vi "邮件发送.vi"(9 "收件人":string, 10 "reference输入":refnum<vi>, 11 "Boolean输入":refnum<vi>) -> ()   [LabVIEW 2016]
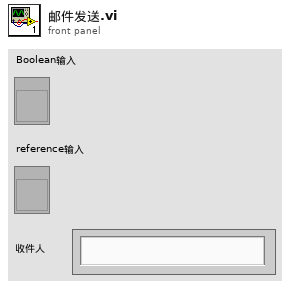
[diagram p1: front panel]
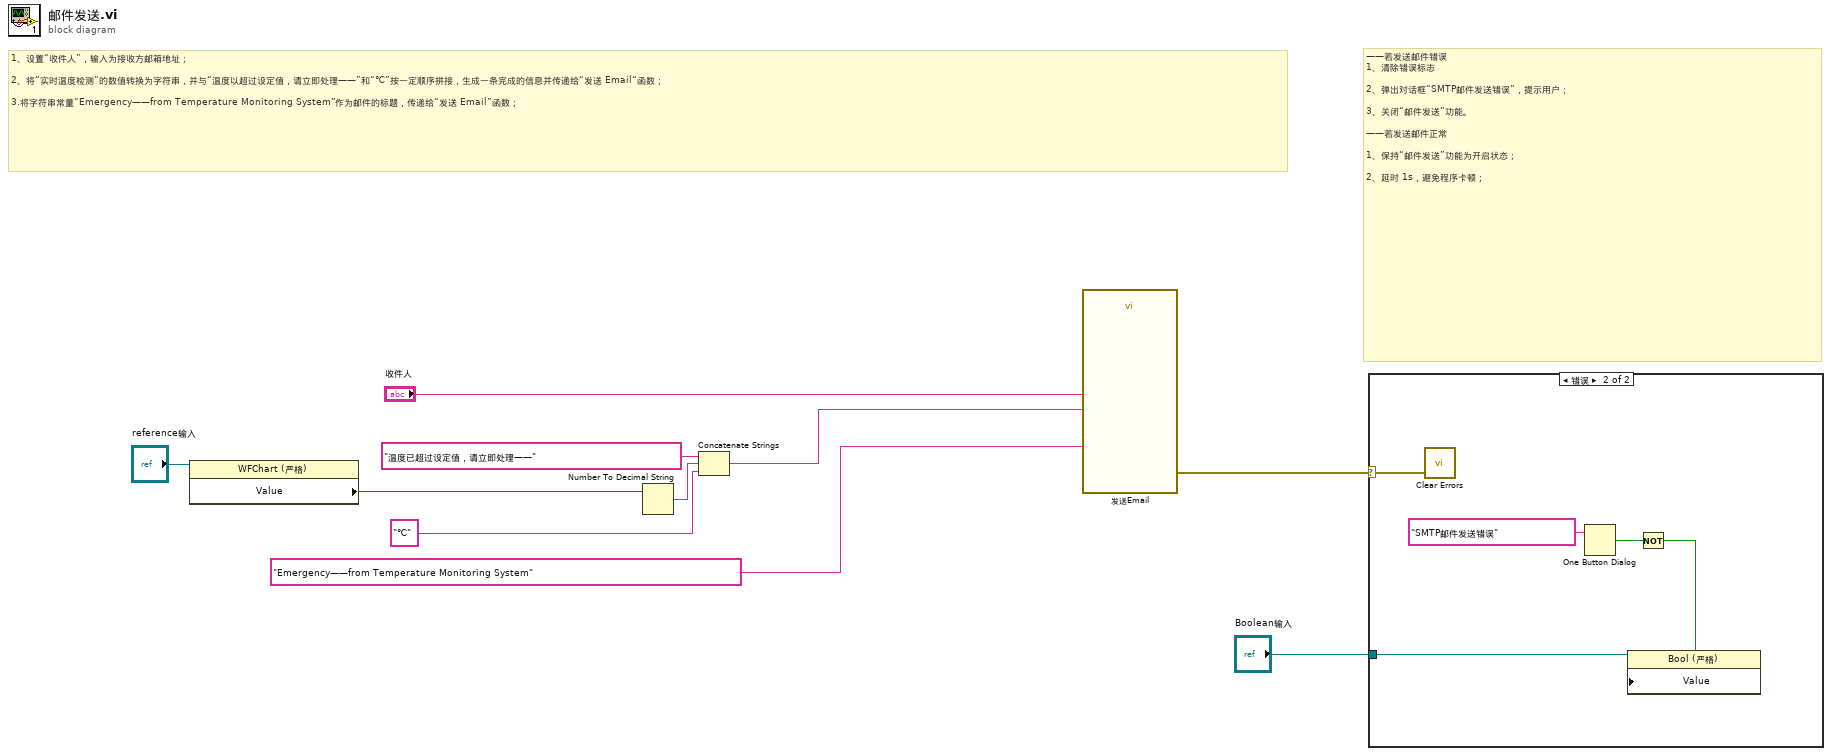
[diagram p0: block diagram]
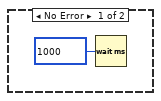
[diagram p2: hidden frame]
diagram:
  # "——若发送邮件错误\n1、清除错误标志\n\n2、弹出对话框“SMTP邮件发送错误”，提示用户；\n\n3、关闭“邮件发送”功能。\n\n——若发送邮件正常\n\n1、保持“邮件发送”功能为开启状态；\n\n2、延时 1s，避免程序卡顿；"
  # "1、设置“收件人”，输入为接收方邮箱地址；\n\n2、将“实时温度检测”的数值转换为字符串，并与“温度以超过设定值，请立即处理——”和“℃”按一定顺序拼接，生成一条完成的信息并传递给“发送 Email“函数；\n\n3.将字符串常量“Emergency——from Temperature Monitoring System”作为邮件的标题，传递给“发送 Email”函数；"
  n1 = property class="WFChart (严格)"(reference="reference输入") -> ("Value"=w1:i32)  [unwired: 1 in, 2 out]
  n2 = Number To Decimal String(number=w1) -> (decimal integer string=w5:string)  [unwired: 1 in]
  n3 = Concatenate Strings("温度已超过设定值，请立即处理——" ("消息"), w5, "℃" ("字符串")) -> (w9:string)
  n4 = call "发送Email"("Message"=w9, "Subject"="Emergency——from Temperature Monitoring System" ("主题"), "Recipients"="收件人") -> ("error out"=w10:errorcluster)  [unwired: 8 in]
  n5 = case shown="错误" w10 {
    selector: w10 -> [_ w12]
    tunnel: "Boolean输入" -> [_ w13]
    frame No Error {
      n6 = Wait (ms)(milliseconds to wait=u32 1000 ("等待时间（毫秒）")) -> ()  [unwired: 1 out]
    }
    frame Error {
      n7 = call <vilib>:"Clear Errors.vi"("error in (no error)"=w12) -> ()  [unwired: 5 in, 2 out]
      n8 = One Button Dialog(message="SMTP邮件发送错误" ("消息")) -> (true=w15:bool)  [unwired: 1 in]
      n9 = Not(x=w15) -> (.not. x?=w14:bool)
      n10 = property class="Bool (严格)"(reference=w13, "Value"=w14) -> ()  [unwired: 1 in, 2 out]
    }
  }
